vi "CODMn字符串显示移位(子VI).vi"(11 "输入字符串":string) -> ()   [LabVIEW 2016, in "斯坦道CODMn.lvlib"]
panel:
  out "校准内容显示输出":string
  in  "停止":bool
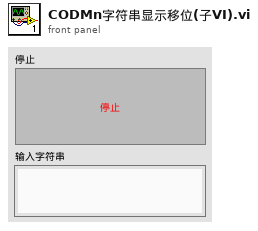
[diagram p1: front panel]
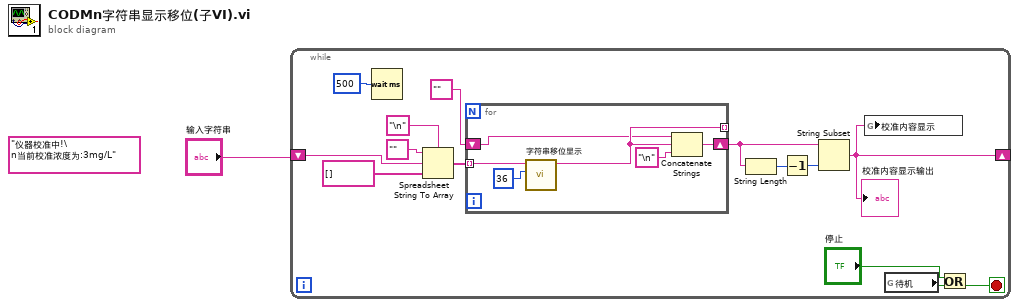
[diagram p0: block diagram]
diagram:
  (unwired) "仪器校准中!\n当前校准浓度为:3mg/L" ("校准内容显示")
  n1 = while {
    shift-right: [w5] -> _
    shift-left: "输入字符串" -> [w10]
    stop <- w3 stop-if-true
    n2 = Wait (ms)(milliseconds to wait=u32 500 ("等待时间（毫秒）")) -> ()  [unwired: 1 out]
    n3 = Spreadsheet String To Array(delimiter (Tab)="\n" ("分隔符(Tab)"), format string="" ("格式字符串"), spreadsheet string=w10, array type (2D Dbl)=string[] []) -> (array=w13:string[])
    n4 = for {
      tunnel: w13 -> [w21] mode=indexing
      tunnel: [w19] -> _ mode=indexing
      shift-right: [w17] -> w8
      shift-left: "" ("格式字符串") -> [w18]
      n5 = call "字符串移位显示.vi"("字符框大小"=36, "字符串输入"=w21) -> ("移位后字符串"=w19:string)  [unwired: 8 in, 1 out]
      n6 = Concatenate Strings(w18, w19, "\n" ("分隔符(Tab)")) -> (w17:string)
    }
    n7 = String Length(string=w8) -> (length=w7:i32)
    n8 = Decrement(x=w7) -> (x-1=w6:i32)
    n9 = String Subset(string=w8, length (rest)=w6) -> (substring=w5:string)  [unwired: 1 in]
    "校准内容显示输出" <- w5
    n10 = global write "COD内部交互全局.vi" "校准内容显示"(w5) -> ()
    n11 = global read "COD内部交互全局.vi" "待机"() -> (w4:bool)
    n12 = Or(x="停止", y=w4) -> (x .or. y?=w3:bool)
  }
